vi "中国方块.vi"() -> ()   [LabVIEW 2013]
uses:
  <vilib>/Utility/inputDevices.llb/keyboardAcquire.vi
panel:
  out "元素":T1(ring)
  out "分数":dbl
  out "保存原速度":dbl
  out "移动方块的最右列":dbl
  out "移动方块的最左列":dbl
  out "重叠方块数目":dbl
  out "界面行数":i32=10
  out "界面列数":i32=10
  out "移动方块的最低行":dbl
  out "下降速度":dbl
  out "列位置":dbl
  out "行位置":dbl
  out "移动后位置信息":dbl[][](array[numeric])
  out "方块位置信息":dbl[][](array[numeric])
  out "随机方块":bool[][](array[boolean])
  out "堆叠后界面":bool[][](array[boolean])
  out "游戏界面":bool[][](array[boolean])
  # "调试界面"
  # "在堆叠后界面显示在游戏界面"
  # "良浩牌游戏机\n童年的最佳选择"
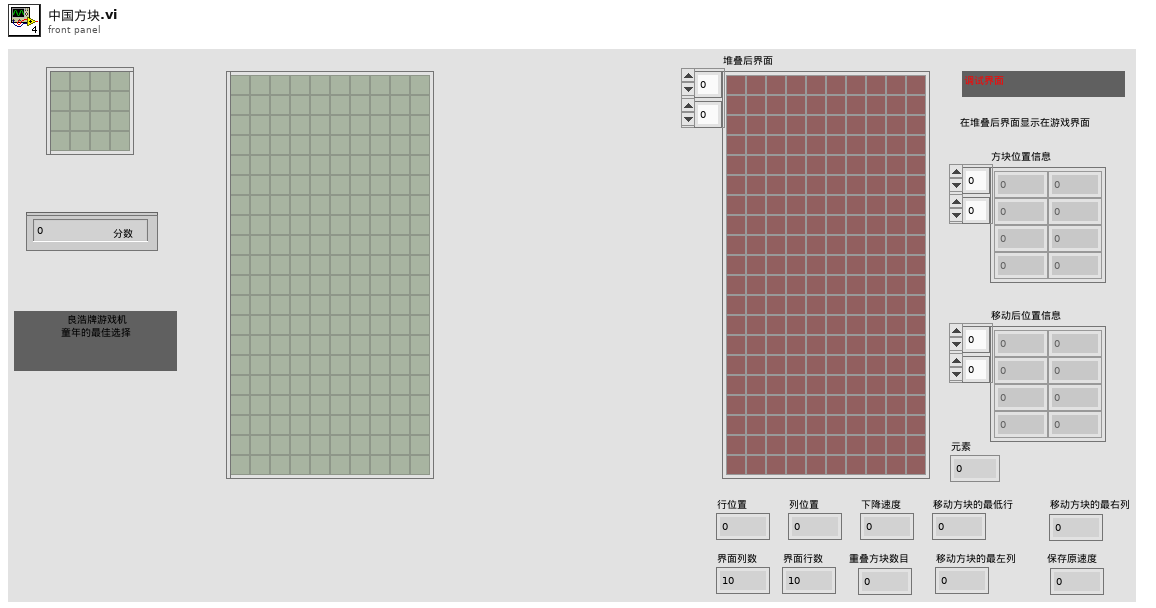
[diagram p1: front panel]
types:
  T1 = enum16{"0", "1", "2", "3", "4", "5", "6", "7", "8", "9", "A", "B", "C", "D", "E", "F", "G", "H", "I", "J", "K", "L", "M", "N", "O", "P", "Q", "R", "S", "T", "U", "V", "W", "X", "Y", "Z", "F1", "F2", "F3", "F4", "F5", "F6", "F7", "F8", "F9", "F10", "F11", "F12", "F13", "F14", "F15", "ADD", "BACK", "BACKSLASH", "CAPITAL", "COMMA", "DECIMAL", "DELETE", "DIVIDE", "DOWN", "END", "EQUALS", "ESCAPE", "GRAVE (`)", "HOME", "INSERT", "LBRACKET", "LCONTROL", "LEFT", "L ALT", "LSHIFT", "LWIN", "MINUS", "MULTIPLY", "NEXT", "NUMLOCK", "NUMPAD_0", "NUMPAD_1", "NUMPAD_2", "NUMPAD_3", "NUMPAD_4", "NUMPAD_5", "NUMPAD_6", "NUMPAD_7", "NUMPAD_8", "NUMPAD_9", "PAUSE", "PERIOD", "PRIOR (PG UP)", "RBRACKET", "RCONTROL", "RETURN", "RIGHT", "R ALT", "RSHIFT", "RWIN", "SCROLL", "SEMICOLON", "SLASH", "SPACE", "SUBTRACT", "TAB", "UP", "ENTER (num pad)", "' (quote)"}
  T2 = enum16{"0", "1", "2", "3", "4", "5", "6", "7", "8", "9", "A", "B", "C", "D", "E", "F", "G", "H", "I", "J", "K", "L", "M", "N", "O", "P", "Q", "R", "S", "T", "U", "V", "W", "X", "Y", "Z", "F1", "F2", "F3", "F4", "F5", "F6", "F7", "F8", "F9", "F10", "F11", "F12", "F13", "F14", "F15", "ADD", "BACK", "BACKSLASH", "CAPITAL", "COMMA", "DECIMAL", "DELETE", "DIVIDE", "DOWN", "END", "EQUALS", "ESCAPE", "GRAVE (`)", "HOME", "INSERT", "LBRACKET", "LCONTROL", "LEFT", "L ALT", "LSHIFT", "LWIN", "MINUS", "MULTIPLY", "NEXT", "NUMLOCK", "NUMPAD_0", "NUMPAD_1", "NUMPAD_2", "NUMPAD_3", "NUMPAD_4", "NUMPAD_5", "NUMPAD_6", "NUMPAD_7", "NUMPAD_8", "NUMPAD_9", "PAUSE", "PERIOD", "PRIOR (PG UP)", "RBRACKET", "RCONTROL", "RETURN", "RIGHT", "R ALT", "RSHIFT", "RWIN", "SCROLL", "SEMICOLON", "SLASH", "SPACE", "SUBTRACT", "TAB", "UP", "ENTER (num pad)", "' (quote)"}[]
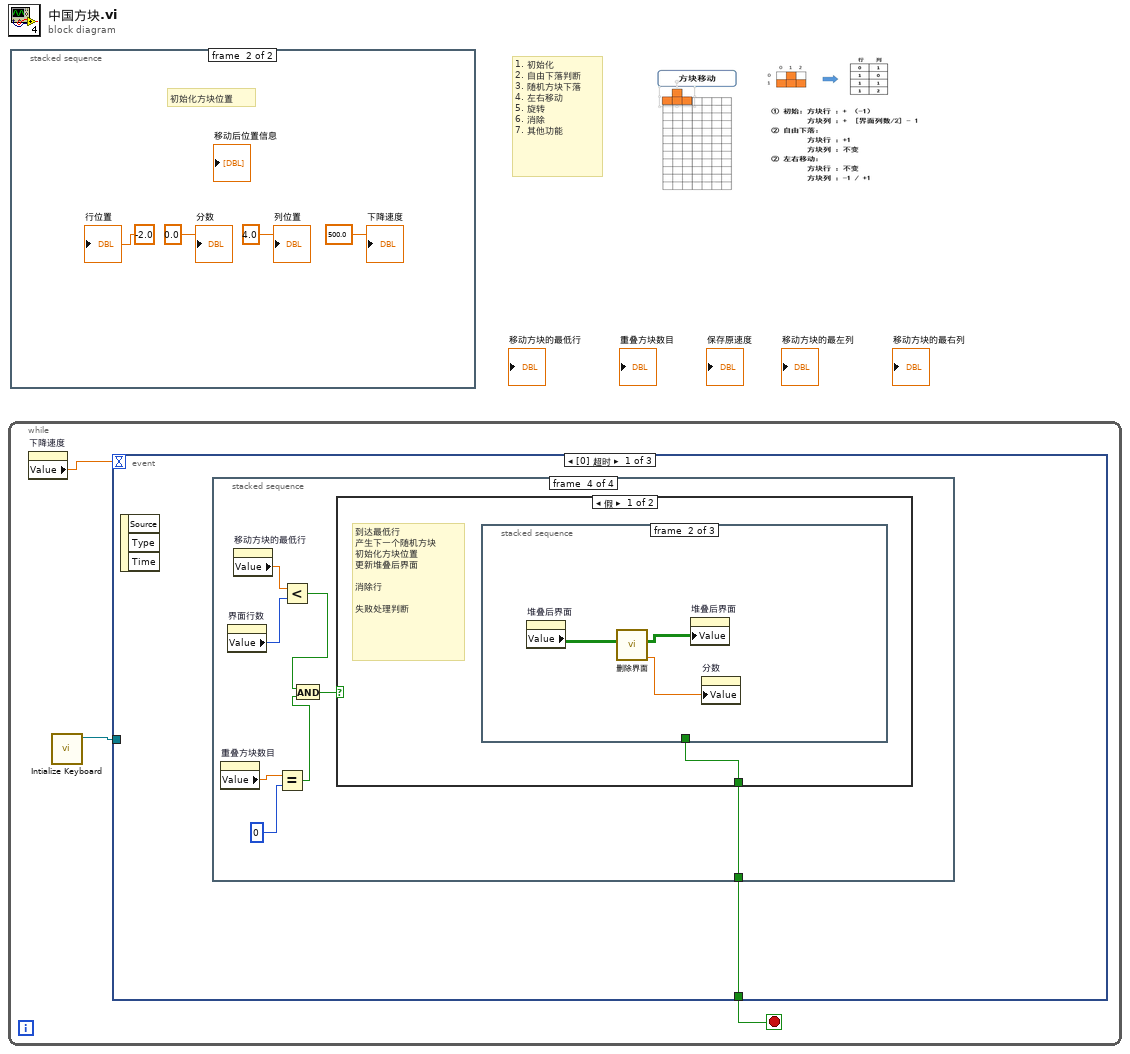
[diagram p0: block diagram]
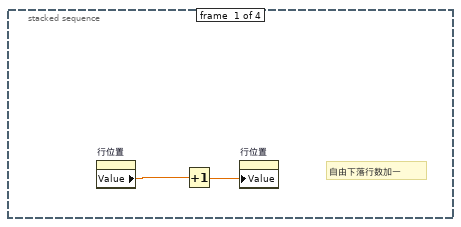
[diagram p2: hidden frame]
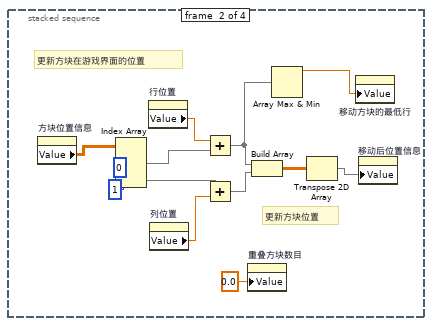
[diagram p3: hidden frame]
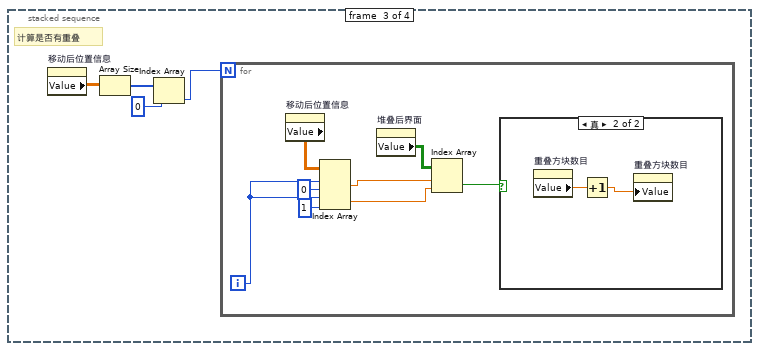
[diagram p4: hidden frame]
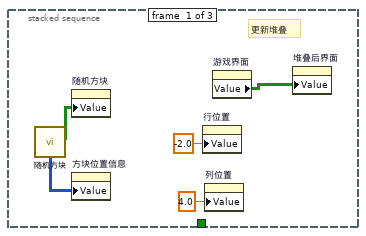
[diagram p6: hidden frame]
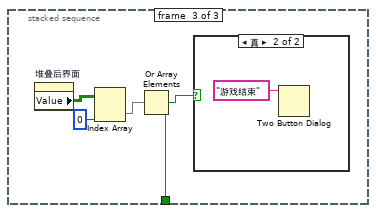
[diagram p7: hidden frame]
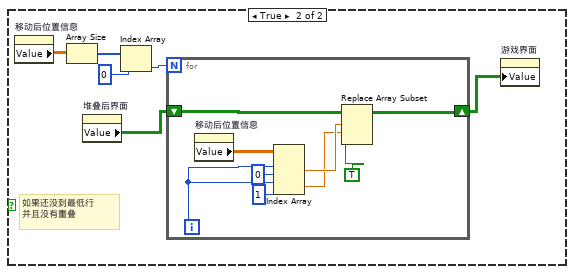
[diagram p9: hidden frame]
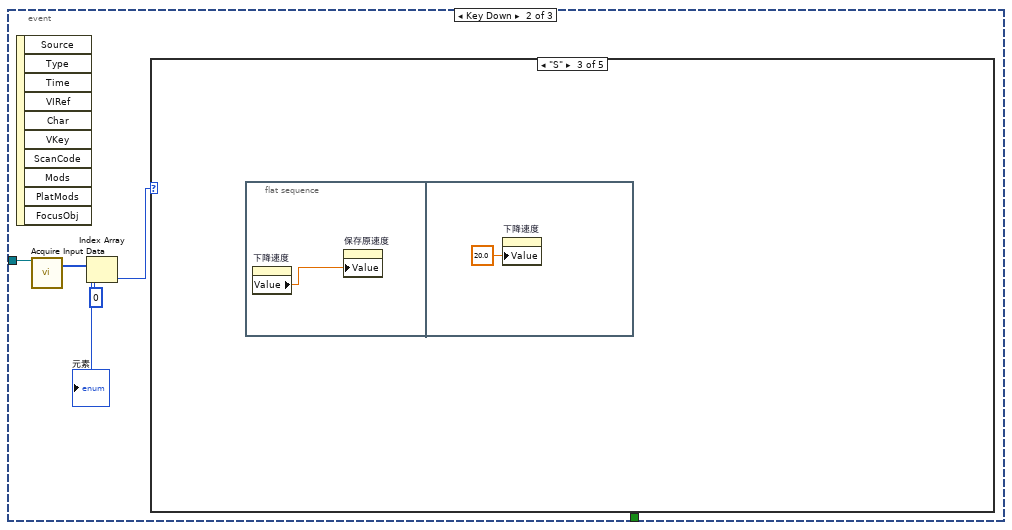
[diagram p10: hidden frame]
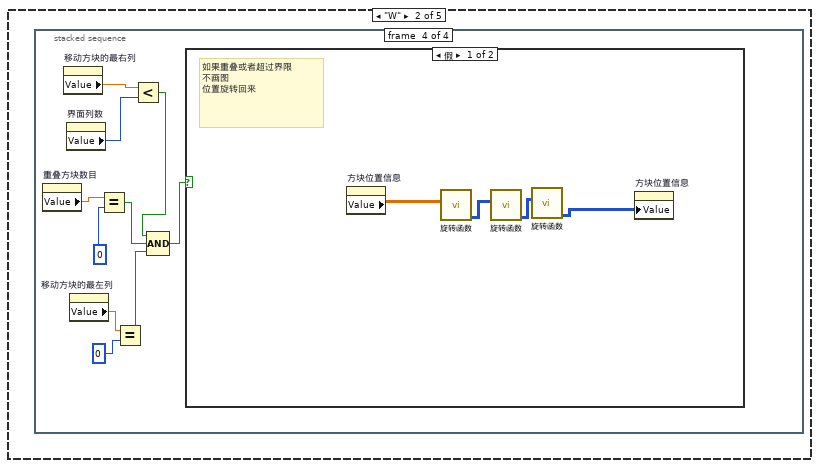
[diagram p12: hidden frame]
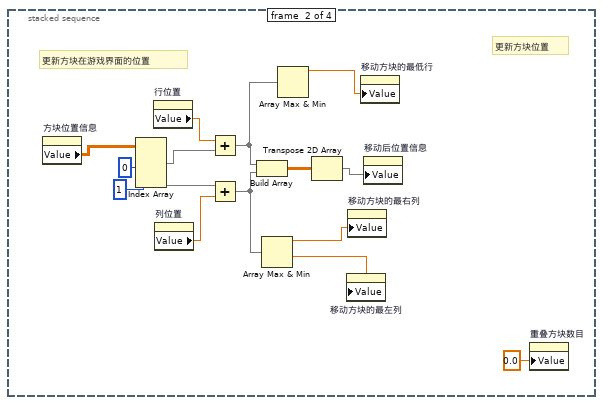
[diagram p14: hidden frame]
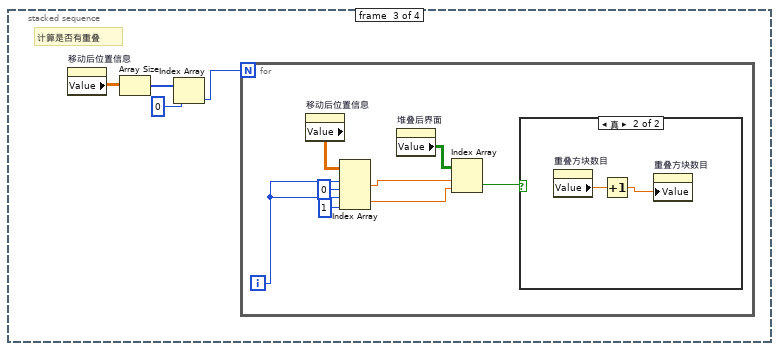
[diagram p15: hidden frame]
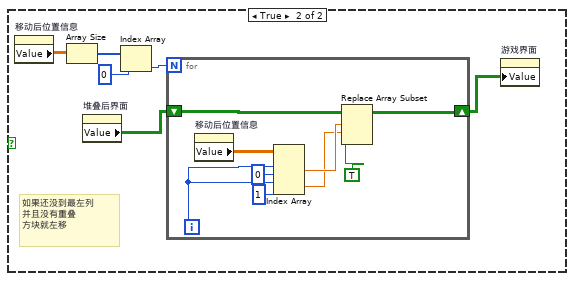
[diagram p17: hidden frame]
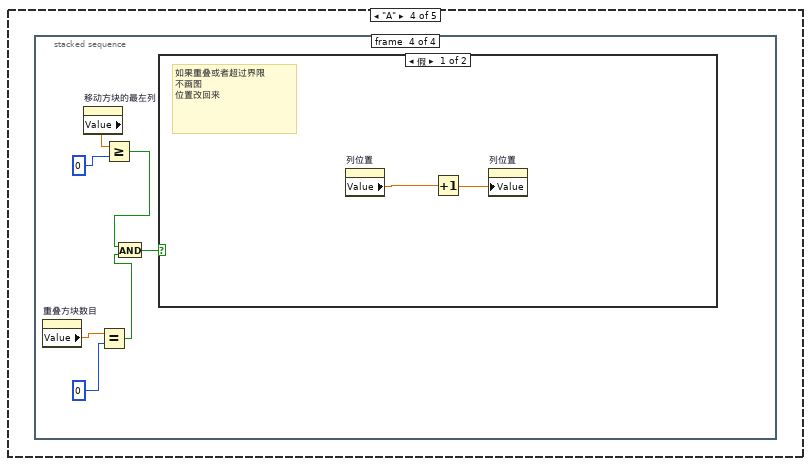
[diagram p18: hidden frame]
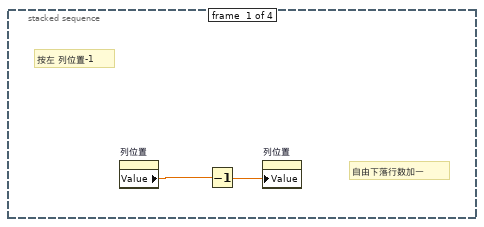
[diagram p19: hidden frame]
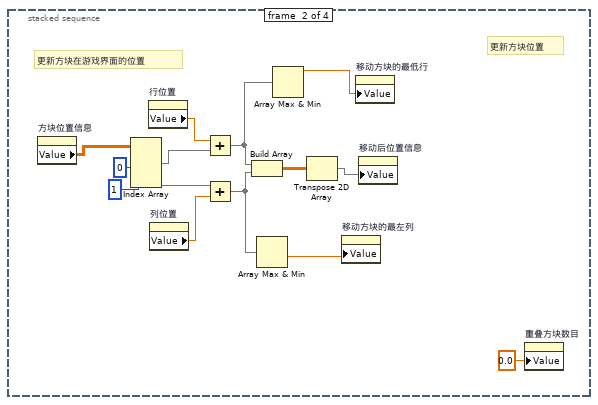
[diagram p20: hidden frame]
diagram:
  # "1. 初始化\n2. 自由下落判断\n3. 随机方块下落\n4. 左右移动\n5. 旋转\n6. 消除\n7. 其他功能"
  n1 = while {
    stop <- w1 stop-if-true
    n2 = property on="下降速度" class="DigNum (严格)"() -> ("Value"=w3:dbl)  [unwired: 2 in, 2 out]
    n3 = call <vilib>:"Intialize Keyboard.vi"() -> ("device ID"=w2:refnum<k1>)  [unwired: 10 in, 1 out]
    n4 = event shown="[0] 超时" {
      selector: _ -> [_ _ _]
      dyn-events: _ -> [_ _ _]
      timeout: w3 -> [_ _ _]
      tunnel: w2 -> [_ w71 _]
      tunnel: [w4 _ _] -> w1
      event Timeout {
        n5 = event-data() -> ()  [unwired: 1 in, 3 out]
        n6 = stacked-sequence {
          tunnel: [_ _ _ w34] -> w4
          frame #0 {
            # "自由下落行数加一"
            n7 = property on="行位置" class="DigNum (严格)"() -> ("Value"=w6:dbl)  [unwired: 2 in, 2 out]
            n8 = Increment(x=w6) -> (x+1=w5:dbl)
            n9 = property on="行位置" class="DigNum (严格)"("Value"=w5) -> ()  [unwired: 2 in, 2 out]
          }
          frame #1 {
            # "更新方块在游戏界面的位置"
            # "更新方块位置"
            n10 = property on="方块位置信息" class="Arr (严格)"() -> ("Value"=w19:dbl[][])  [unwired: 2 in, 2 out]
            n11 = Index Array(array=w19, index (col) #1=0 ("禁用的索引 (列)"), index (col) #2=1 ("索引 (列)")) -> (element #1=w16:dbl[], element #2=w15:dbl[])  [unwired: 2 in]
            n12 = property on="行位置" class="DigNum (严格)"() -> ("Value"=w14:dbl)  [unwired: 2 in, 2 out]
            n13 = property on="列位置" class="DigNum (严格)"() -> ("Value"=w13:dbl)  [unwired: 2 in, 2 out]
            n14 = Add(x=w14, y=w16) -> (x+y=w9:dbl[])
            n15 = Add(x=w15, y=w13) -> (x+y=w12:dbl[])
            n16 = property on="重叠方块数目" class="DigNum (严格)"("Value"=0.0 ("方块的最低行")) -> ()  [unwired: 2 in, 2 out]
            n17 = Build Array(w9, w12) -> (w11:dbl[][])
            n18 = Array Max & Min(array=w9) -> (max value=w8:dbl)  [unwired: 3 out]
            n19 = Transpose 2D Array(2D array=w11) -> (transposed array=w10:dbl[][])
            n20 = property on="移动方块的最低行" class="DigNum (严格)"("Value"=w8) -> ()  [unwired: 2 in, 2 out]
            n21 = property on="移动后位置信息" class="Arr (严格)"("Value"=w10) -> ()  [unwired: 2 in, 2 out]
          }
          frame #2 {
            # "计算是否有重叠"
            n22 = property on="移动后位置信息" class="Arr (严格)"() -> ("Value"=w23:dbl[][])  [unwired: 2 in, 2 out]
            n23 = Array Size(array=w23) -> (size(s)=w22:i32[])
            n24 = Index Array(array=w22, index=0 ("索引")) -> (element=w20:i32)
            n25 = for {
              N: w20 -> [_]
              i -> [w30]
              n26 = property on="移动后位置信息" class="Arr (严格)"() -> ("Value"=w31:dbl[][])  [unwired: 2 in, 2 out]
              n27 = Index Array(array=w31, index (row) #1=w30, index (col) #1=0 ("禁用的索引 (列)"), index (row) #2=w30, index (col) #2=1 ("禁用的索引 (列)")) -> (element #1=w26:dbl, element #2=w25:dbl)
              n28 = property on="堆叠后界面" class="Arr (严格)"() -> ("Value"=w27:bool[][])  [unwired: 2 in, 2 out]
              n29 = Index Array(array=w27, index (row)=w26, index (col)=w25) -> (element=w24:bool)
              n30 = case shown="真" w24 {
                frame False {
                }
                frame True {
                  n31 = property on="重叠方块数目" class="DigNum (严格)"() -> ("Value"=w33:dbl)  [unwired: 2 in, 2 out]
                  n32 = Increment(x=w33) -> (x+1=w32:dbl)
                  n33 = property on="重叠方块数目" class="DigNum (严格)"("Value"=w32) -> ()  [unwired: 2 in, 2 out]
                }
              }
            }
          }
          frame #3 {
            n34 = property on="重叠方块数目" class="DigNum (严格)"() -> ("Value"=w39:dbl)  [unwired: 2 in, 2 out]
            n35 = property on="界面行数" class="DigNum (严格)"() -> ("Value"=w40:i32)  [unwired: 2 in, 2 out]
            n36 = property on="移动方块的最低行" class="DigNum (严格)"() -> ("Value"=w41:dbl)  [unwired: 2 in, 2 out]
            n37 = Equal?(x=w39, y=0) -> (x = y?=w37:bool)
            n38 = Less?(x=w41, y=w40) -> (x < y?=w38:bool)
            n39 = And(x=w38, y=w37) -> (x .and. y?=w36:bool)
            n40 = case shown="假" w36 {
              tunnel: [w42 _] -> w34
              frame False {
                # "到达最低行\n产生下一个随机方块\n初始化方块位置\n更新堆叠后界面\n\n消除行\n\n失败处理判断"
                n41 = stacked-sequence {
                  tunnel: [_ _ w51] -> w42
                  frame #0 {
                    # "更新堆叠"
                    n42 = call "随机方块.vi"() -> ("方块位置信息"=w46:i32[][], "随机方块"=w47:bool[][])  [unwired: 10 in]
                    n43 = property on="随机方块" class="Arr (严格)"("Value"=w47) -> ()  [unwired: 2 in, 2 out]
                    n44 = property on="方块位置信息" class="Arr (严格)"("Value"=w46) -> ()  [unwired: 2 in, 2 out]
                    n45 = property on="行位置" class="DigNum (严格)"("Value"=-2.0 ("行位置")) -> ()  [unwired: 2 in, 2 out]
                    n46 = property on="列位置" class="DigNum (严格)"("Value"=4.0 ("列位置")) -> ()  [unwired: 2 in, 2 out]
                    n47 = property on="游戏界面" class="Arr (严格)"() -> ("Value"=w43:bool[][])  [unwired: 2 in, 2 out]
                    n48 = property on="堆叠后界面" class="Arr (严格)"("Value"=w43) -> ()  [unwired: 2 in, 2 out]
                  }
                  frame #1 {
                    n49 = property on="堆叠后界面" class="Arr (严格)"() -> ("Value"=w50:bool[][])  [unwired: 2 in, 2 out]
                    n50 = call "删除界面.vi"("删除前的界面"=w50) -> ("删除行数"=w48:dbl, "删除后的界面"=w49:bool[][])  [unwired: 9 in]
                    n51 = property on="堆叠后界面" class="Arr (严格)"("Value"=w49) -> ()  [unwired: 2 in, 2 out]
                    n52 = property on="分数" class="DigNum (严格)"("Value"=w48) -> ()  [unwired: 2 in, 2 out]
                  }
                  frame #2 {
                    n53 = property on="堆叠后界面" class="Arr (严格)"() -> ("Value"=w54:bool[][])  [unwired: 2 in, 2 out]
                    n54 = Index Array(array=w54, index (row)=0 ("索引 (行)")) -> (element=w52:bool[])  [unwired: 1 in]
                    n55 = Or Array Elements(Boolean array=w52) -> (logical OR=w51:bool)
                    n56 = case shown="真" w51 {
                      frame False {
                      }
                      frame True {
                        n57 = Two Button Dialog(message="游戏结束" ("消息")) -> ()  [unwired: 2 in, 1 out]
                      }
                    }
                  }
                }
              }
              frame True {
                # "如果还没到最低行\n并且没有重叠"
                n58 = property on="移动后位置信息" class="Arr (严格)"() -> ("Value"=w61:dbl[][])  [unwired: 2 in, 2 out]
                n59 = Array Size(array=w61) -> (size(s)=w60:i32[])
                n60 = property on="堆叠后界面" class="Arr (严格)"() -> ("Value"=w57:bool[][])  [unwired: 2 in, 2 out]
                n61 = Index Array(array=w60, index=0 ("索引")) -> (element=w58:i32)
                n62 = for {
                  N: w58 -> [_]
                  shift-right: [w65] -> w56
                  shift-left: w57 -> [w66]
                  i -> [w69]
                  n63 = property on="移动后位置信息" class="Arr (严格)"() -> ("Value"=w70:dbl[][])  [unwired: 2 in, 2 out]
                  n64 = Index Array(array=w70, index (row) #1=w69, index (col) #1=0 ("禁用的索引 (列)"), index (row) #2=w69, index (col) #2=1 ("禁用的索引 (列)")) -> (element #1=w64:dbl, element #2=w63:dbl)
                  n65 = Replace Array Subset(array=w66, new element=TRUE, index (row)=w64, index (col)=w63) -> (w65:bool[][])
                }
                n66 = property on="游戏界面" class="Arr (严格)"("Value"=w56) -> ()  [unwired: 2 in, 2 out]
              }
            }
          }
        }
      }
      event Key Down {
        n67 = event-data() -> ()  [unwired: 1 in, 10 out]
        n68 = call-poly <vilib>:"Acquire Input Data.vi"("device ID"=w71) -> ("keys pressed"=w74:T2)  [unwired: 16 in, 2 out]
        n69 = Index Array(array=w74, index=0 ("索引")) -> (element=w72:T1)
        "元素" <- w72
        n70 = case shown="\"S\"" w72 {
          frame "0", Default {
          }
          frame "W" {
            n71 = stacked-sequence {
              frame #0 {
                # "按上旋转"
              }
              frame #1 {
                # "更新方块在游戏界面的位置"
                # "更新方块位置"
                n72 = property on="方块位置信息" class="Arr (严格)"() -> ("Value"=w89:dbl[][])  [unwired: 2 in, 2 out]
                n73 = Index Array(array=w89, index (col) #1=0 ("禁用的索引 (列)"), index (col) #2=1 ("索引 (列)")) -> (element #1=w86:dbl[], element #2=w85:dbl[])  [unwired: 2 in]
                n74 = property on="行位置" class="DigNum (严格)"() -> ("Value"=w84:dbl)  [unwired: 2 in, 2 out]
                n75 = property on="列位置" class="DigNum (严格)"() -> ("Value"=w83:dbl)  [unwired: 2 in, 2 out]
                n76 = Add(x=w84, y=w86) -> (x+y=w80:dbl[])
                n77 = Add(x=w85, y=w83) -> (x+y=w77:dbl[])
                n78 = Build Array(w80, w77) -> (w82:dbl[][])
                n79 = Array Max & Min(array=w77) -> (max value=w75:dbl, min value=w76:dbl)  [unwired: 2 out]
                n80 = Array Max & Min(array=w80) -> (max value=w79:dbl)  [unwired: 3 out]
                n81 = Transpose 2D Array(2D array=w82) -> (transposed array=w81:dbl[][])
                n82 = property on="移动方块的最左列" class="DigNum (严格)"("Value"=w76) -> ()  [unwired: 2 in, 2 out]
                n83 = property on="移动方块的最右列" class="DigNum (严格)"("Value"=w75) -> ()  [unwired: 2 in, 2 out]
                n84 = property on="移动方块的最低行" class="DigNum (严格)"("Value"=w79) -> ()  [unwired: 2 in, 2 out]
                n85 = property on="移动后位置信息" class="Arr (严格)"("Value"=w81) -> ()  [unwired: 2 in, 2 out]
                n86 = property on="重叠方块数目" class="DigNum (严格)"("Value"=0.0 ("方块的最低行")) -> ()  [unwired: 2 in, 2 out]
              }
              frame #2 {
                # "计算是否有重叠"
                n87 = property on="移动后位置信息" class="Arr (严格)"() -> ("Value"=w93:dbl[][])  [unwired: 2 in, 2 out]
                n88 = Array Size(array=w93) -> (size(s)=w92:i32[])
                n89 = Index Array(array=w92, index=0 ("索引")) -> (element=w90:i32)
                n90 = for {
                  N: w90 -> [_]
                  i -> [w100]
                  n91 = property on="移动后位置信息" class="Arr (严格)"() -> ("Value"=w101:dbl[][])  [unwired: 2 in, 2 out]
                  n92 = Index Array(array=w101, index (row) #1=w100, index (col) #1=0 ("禁用的索引 (列)"), index (row) #2=w100, index (col) #2=1 ("禁用的索引 (列)")) -> (element #1=w96:dbl, element #2=w95:dbl)
                  n93 = property on="堆叠后界面" class="Arr (严格)"() -> ("Value"=w97:bool[][])  [unwired: 2 in, 2 out]
                  n94 = Index Array(array=w97, index (row)=w96, index (col)=w95) -> (element=w94:bool)
                  n95 = case shown="真" w94 {
                    frame False {
                    }
                    frame True {
                      n96 = property on="重叠方块数目" class="DigNum (严格)"() -> ("Value"=w103:dbl)  [unwired: 2 in, 2 out]
                      n97 = Increment(x=w103) -> (x+1=w102:dbl)
                      n98 = property on="重叠方块数目" class="DigNum (严格)"("Value"=w102) -> ()  [unwired: 2 in, 2 out]
                    }
                  }
                }
              }
              frame #3 {
                n99 = property on="重叠方块数目" class="DigNum (严格)"() -> ("Value"=w112:dbl)  [unwired: 2 in, 2 out]
                n100 = property on="移动方块的最右列" class="DigNum (严格)"() -> ("Value"=w113:dbl)  [unwired: 2 in, 2 out]
                n101 = property on="界面列数" class="DigNum (严格)"() -> ("Value"=w110:i32)  [unwired: 2 in, 2 out]
                n102 = property on="移动方块的最左列" class="DigNum (严格)"() -> ("Value"=w106:dbl)  [unwired: 2 in, 2 out]
                n103 = Equal?(x=w112, y=0) -> (x = y?=w108:bool)
                n104 = Equal?(x=w106, y=0) -> (x = y?=w109:bool)
                n105 = Less?(x=w113, y=w110) -> (x < y?=w107:bool)
                n106 = Compound Arithmetic op=AND(w107, w108, w109) -> (w104:bool)
                n107 = case shown="假" w104 {
                  frame False {
                    # "如果重叠或者超过界限\n不画图\n位置旋转回来"
                    n108 = property on="方块位置信息" class="Arr (严格)"() -> ("Value"=w117:dbl[][])  [unwired: 2 in, 2 out]
                    n109 = call "旋转函数.vi"("原始方块位置"=w117) -> ("旋转方块位置"=w116:i32[][])  [unwired: 9 in, 1 out]
                    n110 = call "旋转函数.vi"("原始方块位置"=w116) -> ("旋转方块位置"=w115:i32[][])  [unwired: 9 in, 1 out]
                    n111 = call "旋转函数.vi"("原始方块位置"=w115) -> ("旋转方块位置"=w114:i32[][])  [unwired: 9 in, 1 out]
                    n112 = property on="方块位置信息" class="Arr (严格)"("Value"=w114) -> ()  [unwired: 2 in, 2 out]
                  }
                  frame True {
                    # "如果还没到最左列\n并且没有重叠\n方块就左移"
                    n113 = property on="移动后位置信息" class="Arr (严格)"() -> ("Value"=w123:dbl[][])  [unwired: 2 in, 2 out]
                    n114 = Array Size(array=w123) -> (size(s)=w122:i32[])
                    n115 = property on="堆叠后界面" class="Arr (严格)"() -> ("Value"=w119:bool[][])  [unwired: 2 in, 2 out]
                    n116 = Index Array(array=w122, index=0 ("索引")) -> (element=w120:i32)
                    n117 = for {
                      N: w120 -> [_]
                      shift-right: [w127] -> w118
                      shift-left: w119 -> [w128]
                      i -> [w131]
                      n118 = property on="移动后位置信息" class="Arr (严格)"() -> ("Value"=w132:dbl[][])  [unwired: 2 in, 2 out]
                      n119 = Index Array(array=w132, index (row) #1=w131, index (col) #1=0 ("禁用的索引 (列)"), index (row) #2=w131, index (col) #2=1 ("禁用的索引 (列)")) -> (element #1=w126:dbl, element #2=w125:dbl)
                      n120 = Replace Array Subset(array=w128, new element=TRUE, index (row)=w126, index (col)=w125) -> (w127:bool[][])
                    }
                    n121 = property on="游戏界面" class="Arr (严格)"("Value"=w118) -> ()  [unwired: 2 in, 2 out]
                  }
                }
              }
            }
          }
          frame "S" {
            n122 = flat-sequence {
              frame #0 {
                n123 = property on="下降速度" class="DigNum (严格)"() -> ("Value"=w133:dbl)  [unwired: 2 in, 2 out]
                n124 = property on="保存原速度" class="DigNum (严格)"("Value"=w133) -> ()  [unwired: 2 in, 2 out]
              }
              frame #1 {
                n125 = property on="下降速度" class="DigNum (严格)"("Value"=20.0 ("下降速度")) -> ()  [unwired: 2 in, 2 out]
              }
            }
          }
          frame "A" {
            n126 = stacked-sequence {
              frame #0 {
                # "按左 列位置-1"
                # "自由下落行数加一"
                n127 = property on="列位置" class="DigNum (严格)"() -> ("Value"=w136:dbl)  [unwired: 2 in, 2 out]
                n128 = Decrement(x=w136) -> (x-1=w135:dbl)
                n129 = property on="列位置" class="DigNum (严格)"("Value"=w135) -> ()  [unwired: 2 in, 2 out]
              }
              frame #1 {
                # "更新方块在游戏界面的位置"
                # "更新方块位置"
                n130 = property on="方块位置信息" class="Arr (严格)"() -> ("Value"=w150:dbl[][])  [unwired: 2 in, 2 out]
                n131 = Index Array(array=w150, index (col) #1=0 ("禁用的索引 (列)"), index (col) #2=1 ("索引 (列)")) -> (element #1=w147:dbl[], element #2=w146:dbl[])  [unwired: 2 in]
                n132 = property on="行位置" class="DigNum (严格)"() -> ("Value"=w145:dbl)  [unwired: 2 in, 2 out]
                n133 = property on="列位置" class="DigNum (严格)"() -> ("Value"=w144:dbl)  [unwired: 2 in, 2 out]
                n134 = Add(x=w145, y=w147) -> (x+y=w141:dbl[])
                n135 = Add(x=w146, y=w144) -> (x+y=w138:dbl[])
                n136 = Build Array(w141, w138) -> (w143:dbl[][])
                n137 = Array Max & Min(array=w138) -> (min value=w137:dbl)  [unwired: 3 out]
                n138 = Array Max & Min(array=w141) -> (max value=w140:dbl)  [unwired: 3 out]
                n139 = Transpose 2D Array(2D array=w143) -> (transposed array=w142:dbl[][])
                n140 = property on="移动方块的最左列" class="DigNum (严格)"("Value"=w137) -> ()  [unwired: 2 in, 2 out]
                n141 = property on="移动方块的最低行" class="DigNum (严格)"("Value"=w140) -> ()  [unwired: 2 in, 2 out]
                n142 = property on="移动后位置信息" class="Arr (严格)"("Value"=w142) -> ()  [unwired: 2 in, 2 out]
                n143 = property on="重叠方块数目" class="DigNum (严格)"("Value"=0.0 ("方块的最低行")) -> ()  [unwired: 2 in, 2 out]
              }
              frame #2 {
                # "计算是否有重叠"
                n144 = property on="移动后位置信息" class="Arr (严格)"() -> ("Value"=w154:dbl[][])  [unwired: 2 in, 2 out]
                n145 = Array Size(array=w154) -> (size(s)=w153:i32[])
                n146 = Index Array(array=w153, index=0 ("索引")) -> (element=w151:i32)
                n147 = for {
                  N: w151 -> [_]
                  i -> [w161]
                  n148 = property on="移动后位置信息" class="Arr (严格)"() -> ("Value"=w162:dbl[][])  [unwired: 2 in, 2 out]
                  n149 = Index Array(array=w162, index (row) #1=w161, index (col) #1=0 ("禁用的索引 (列)"), index (row) #2=w161, index (col) #2=1 ("禁用的索引 (列)")) -> (element #1=w157:dbl, element #2=w156:dbl)
                  n150 = property on="堆叠后界面" class="Arr (严格)"() -> ("Value"=w158:bool[][])  [unwired: 2 in, 2 out]
                  n151 = Index Array(array=w158, index (row)=w157, index (col)=w156) -> (element=w155:bool)
                  n152 = case shown="真" w155 {
                    frame False {
                    }
                    frame True {
                      n153 = property on="重叠方块数目" class="DigNum (严格)"() -> ("Value"=w164:dbl)  [unwired: 2 in, 2 out]
                      n154 = Increment(x=w164) -> (x+1=w163:dbl)
                      n155 = property on="重叠方块数目" class="DigNum (严格)"("Value"=w163) -> ()  [unwired: 2 in, 2 out]
                    }
                  }
                }
              }
              frame #3 {
                n156 = property on="重叠方块数目" class="DigNum (严格)"() -> ("Value"=w170:dbl)  [unwired: 2 in, 2 out]
                n157 = property on="移动方块的最左列" class="DigNum (严格)"() -> ("Value"=w171:dbl)  [unwired: 2 in, 2 out]
                n158 = Equal?(x=w170, y=0) -> (x = y?=w168:bool)
                n159 = Greater Or Equal?(x=w171, y=0) -> (x >= y?=w169:bool)
                n160 = And(x=w169, y=w168) -> (x .and. y?=w167:bool)
                n161 = case shown="假" w167 {
                  frame False {
                    # "如果重叠或者超过界限\n不画图\n位置改回来"
                    n162 = property on="列位置" class="DigNum (严格)"() -> ("Value"=w173:dbl)  [unwired: 2 in, 2 out]
                    n163 = Increment(x=w173) -> (x+1=w172:dbl)
                    n164 = property on="列位置" class="DigNum (严格)"("Value"=w172) -> ()  [unwired: 2 in, 2 out]
                  }
                  frame True {
                    # "如果还没到最左列\n并且没有重叠\n方块就左移"
                    n165 = property on="移动后位置信息" class="Arr (严格)"() -> ("Value"=w179:dbl[][])  [unwired: 2 in, 2 out]
                    n166 = Array Size(array=w179) -> (size(s)=w178:i32[])
                    n167 = property on="堆叠后界面" class="Arr (严格)"() -> ("Value"=w175:bool[][])  [unwired: 2 in, 2 out]
                    n168 = Index Array(array=w178, index=0 ("索引")) -> (element=w176:i32)
                    n169 = for {
                      N: w176 -> [_]
                      shift-right: [w183] -> w174
                      shift-left: w175 -> [w184]
                      i -> [w187]
                      n170 = property on="移动后位置信息" class="Arr (严格)"() -> ("Value"=w188:dbl[][])  [unwired: 2 in, 2 out]
                      n171 = Index Array(array=w188, index (row) #1=w187, index (col) #1=0 ("禁用的索引 (列)"), index (row) #2=w187, index (col) #2=1 ("禁用的索引 (列)")) -> (element #1=w182:dbl, element #2=w181:dbl)
                      n172 = Replace Array Subset(array=w184, new element=TRUE, index (row)=w182, index (col)=w181) -> (w183:bool[][])
                    }
                    n173 = property on="游戏界面" class="Arr (严格)"("Value"=w174) -> ()  [unwired: 2 in, 2 out]
                  }
                }
              }
            }
          }
          frame "D" {
            n174 = stacked-sequence {
              frame #0 {
                # "按右 列位置+1"
                # "自由下落行数加一"
                n175 = property on="列位置" class="DigNum (严格)"() -> ("Value"=w190:dbl)  [unwired: 2 in, 2 out]
                n176 = Increment(x=w190) -> (x+1=w189:dbl)
                n177 = property on="列位置" class="DigNum (严格)"("Value"=w189) -> ()  [unwired: 2 in, 2 out]
              }
              frame #1 {
                # "更新方块在游戏界面的位置"
                # "更新方块位置"
                n178 = property on="方块位置信息" class="Arr (严格)"() -> ("Value"=w205:dbl[][])  [unwired: 2 in, 2 out]
                n179 = Index Array(array=w205, index (col) #1=0 ("禁用的索引 (列)"), index (col) #2=1 ("索引 (列)")) -> (element #1=w202:dbl[], element #2=w201:dbl[])  [unwired: 2 in]
                n180 = property on="行位置" class="DigNum (严格)"() -> ("Value"=w200:dbl)  [unwired: 2 in, 2 out]
                n181 = property on="列位置" class="DigNum (严格)"() -> ("Value"=w199:dbl)  [unwired: 2 in, 2 out]
                n182 = Add(x=w200, y=w202) -> (x+y=w196:dbl[])
                n183 = Add(x=w201, y=w199) -> (x+y=w193:dbl[])
                n184 = Build Array(w196, w193) -> (w198:dbl[][])
                n185 = Array Max & Min(array=w193) -> (max value=w191:dbl, min value=w192:dbl)  [unwired: 2 out]
                n186 = Array Max & Min(array=w196) -> (max value=w195:dbl)  [unwired: 3 out]
                n187 = Transpose 2D Array(2D array=w198) -> (transposed array=w197:dbl[][])
                n188 = property on="移动方块的最左列" class="DigNum (严格)"("Value"=w192) -> ()  [unwired: 2 in, 2 out]
                n189 = property on="移动方块的最右列" class="DigNum (严格)"("Value"=w191) -> ()  [unwired: 2 in, 2 out]
                n190 = property on="移动方块的最低行" class="DigNum (严格)"("Value"=w195) -> ()  [unwired: 2 in, 2 out]
                n191 = property on="移动后位置信息" class="Arr (严格)"("Value"=w197) -> ()  [unwired: 2 in, 2 out]
                n192 = property on="重叠方块数目" class="DigNum (严格)"("Value"=0.0 ("方块的最低行")) -> ()  [unwired: 2 in, 2 out]
              }
              frame #2 {
                # "计算是否有重叠"
                n193 = property on="移动后位置信息" class="Arr (严格)"() -> ("Value"=w209:dbl[][])  [unwired: 2 in, 2 out]
                n194 = Array Size(array=w209) -> (size(s)=w208:i32[])
                n195 = Index Array(array=w208, index=0 ("索引")) -> (element=w206:i32)
                n196 = for {
                  N: w206 -> [_]
                  i -> [w216]
                  n197 = property on="移动后位置信息" class="Arr (严格)"() -> ("Value"=w217:dbl[][])  [unwired: 2 in, 2 out]
                  n198 = Index Array(array=w217, index (row) #1=w216, index (col) #1=0 ("禁用的索引 (列)"), index (row) #2=w216, index (col) #2=1 ("禁用的索引 (列)")) -> (element #1=w212:dbl, element #2=w211:dbl)
                  n199 = property on="堆叠后界面" class="Arr (严格)"() -> ("Value"=w213:bool[][])  [unwired: 2 in, 2 out]
                  n200 = Index Array(array=w213, index (row)=w212, index (col)=w211) -> (element=w210:bool)
                  n201 = case shown="真" w210 {
                    frame False {
                    }
                    frame True {
                      n202 = property on="重叠方块数目" class="DigNum (严格)"() -> ("Value"=w219:dbl)  [unwired: 2 in, 2 out]
                      n203 = Increment(x=w219) -> (x+1=w218:dbl)
                      n204 = property on="重叠方块数目" class="DigNum (严格)"("Value"=w218) -> ()  [unwired: 2 in, 2 out]
                    }
                  }
                }
              }
              frame #3 {
                n205 = property on="移动方块的最右列" class="DigNum (严格)"() -> ("Value"=w226:dbl)  [unwired: 2 in, 2 out]
                n206 = property on="重叠方块数目" class="DigNum (严格)"() -> ("Value"=w225:dbl)  [unwired: 2 in, 2 out]
                n207 = property on="界面列数" class="DigNum (严格)"() -> ("Value"=w220:i32)  [unwired: 2 in, 2 out]
                n208 = Equal?(x=w225, y=0) -> (x = y?=w223:bool)
                n209 = Less?(x=w226, y=w220) -> (x < y?=w224:bool)
                n210 = And(x=w224, y=w223) -> (x .and. y?=w222:bool)
                n211 = case shown="假" w222 {
                  frame False {
                    # "如果重叠或者超过界限\n不画图\n位置改回来"
                    n212 = property on="列位置" class="DigNum (严格)"() -> ("Value"=w228:dbl)  [unwired: 2 in, 2 out]
                    n213 = Decrement(x=w228) -> (x-1=w227:dbl)
                    n214 = property on="列位置" class="DigNum (严格)"("Value"=w227) -> ()  [unwired: 2 in, 2 out]
                  }
                  frame True {
                    # "如果还没到最左列\n并且没有重叠\n方块就左移"
                    n215 = property on="移动后位置信息" class="Arr (严格)"() -> ("Value"=w234:dbl[][])  [unwired: 2 in, 2 out]
                    n216 = Array Size(array=w234) -> (size(s)=w233:i32[])
                    n217 = property on="堆叠后界面" class="Arr (严格)"() -> ("Value"=w230:bool[][])  [unwired: 2 in, 2 out]
                    n218 = Index Array(array=w233, index=0 ("索引")) -> (element=w231:i32)
                    n219 = for {
                      N: w231 -> [_]
                      shift-right: [w238] -> w229
                      shift-left: w230 -> [w239]
                      i -> [w242]
                      n220 = property on="移动后位置信息" class="Arr (严格)"() -> ("Value"=w243:dbl[][])  [unwired: 2 in, 2 out]
                      n221 = Index Array(array=w243, index (row) #1=w242, index (col) #1=0 ("禁用的索引 (列)"), index (row) #2=w242, index (col) #2=1 ("禁用的索引 (列)")) -> (element #1=w237:dbl, element #2=w236:dbl)
                      n222 = Replace Array Subset(array=w239, new element=TRUE, index (row)=w237, index (col)=w236) -> (w238:bool[][])
                    }
                    n223 = property on="游戏界面" class="Arr (严格)"("Value"=w229) -> ()  [unwired: 2 in, 2 out]
                  }
                }
              }
            }
          }
        }
      }
      event Key Up {
        # "恢复原始速度"
        n224 = event-data() -> ()  [unwired: 1 in, 8 out]
        n225 = property on="保存原速度" class="DigNum (严格)"() -> ("Value"=w244:dbl)  [unwired: 2 in, 2 out]
        n226 = property on="下降速度" class="DigNum (严格)"("Value"=w244) -> ()  [unwired: 2 in, 2 out]
      }
    }
  }
  n227 = stacked-sequence {
    frame #0 {
      w249 = 10 ("维数大小")
      w245 = 20 ("维数大小")
      # "初始化方块"
      # "初始化数组"
      n228 = Initialize Array(FALSE, w245, w249) -> (→"游戏界面" →"堆叠后界面":bool[][])
      n229 = call "随机方块.vi"() -> ("方块位置信息"=→"方块位置信息":i32[][], "随机方块"=→"随机方块":bool[][])  [unwired: 10 in]
      "界面列数" <- w249
      "界面行数" <- w245
    }
    frame #1 {
      # "初始化方块位置"
      "行位置" <- -2.0 ("行位置")
      "列位置" <- 4.0 ("列位置")
      "下降速度" <- 500.0 ("下降速度")
      "分数" <- 0.0 ("分数")
    }
  }
